vi "MarkedRobot.vi"(9 "id":u32, 10 "IA State Input":T2={"our_robots"=[], "enemy_robots"=[], "balls"=[], "geometry"={"line_width"=0, "field_length"=0, "field_width"=0, "boundary_width"=0, "referee_width"=0, "goal_width"=0, "goal_depth"=0, "goal_wall_width"=0, "center_circle_radius"=0, "defense_radius"=0, "defense_stretch"=0, "free_kick_from_defense_dist"=0, "penalty_spot_from_field_line_dist"=0, "penalty_line_from_spot_dist"=0}, "IA Judge"={"stage"="", "command"="", "our_goalie_id"=0.0, "enemy_goalie_id"=0.0, "command enum"=enum."Halt", "Time"=enum."Azul"}, "Received Timestamp"=timestamp(0 s since 1904-01-01), "Events"={"Touch"=FALSE, "Ball out"=FALSE, "id touch"=0.0, "Ball out of \nVision"=FALSE, "Ball inside \nGoalie area"=FALSE, "Robot not responding"=FALSE, "Robots responding status"=[1.0, 1.0, 1.0, 1.0, 1.0, 1.0], "Enemy Ball \nPossession"=FALSE, "Pass State"=FALSE, "id end of pass"=0.0, "Kick"=FALSE, "Id ini Possession"=0.0, "Ball Possesion"=FALSE, "Id Possesion"=0.0, "Direct Kick"=FALSE, "2nd Strk Ativo"=FALSE}}, 11 "AI Parameters":T1={"GotoKick"={"Dist do cone a frente"=150.0, "attacker farback"=1500.0, "Perto"=300.0, "min dist to kick"=150.0, "kick eps"=0.0, "Time to transition"=0.05}, "Attacker"={"CC chute"=0.09, "CC passe"=0.045, "Kick Force"=100.0, "ball-robot Kick"=200.0, "ball-robot Pass"=0.3, "drible\nAttk"=FALSE}, "Defender"={"D max"=1700.0, "Vel p/ robô av"=1000.0, "Kick Force"=100.0, "D atk-def"=0.0, "D farback"=0.0, "drible\ndef"=FALSE, "drible\ngoalie"=FALSE}, "Timeout"={"Field/v in x"=6.0, "Dist Robots"=300, "Dist up in y"=300}, "Pose Striker"={"dist"=200.0, "Numeric"=-4.0, "dist 2"=200.0, "drible\nstriker"=FALSE}, "Dist Stop"=300.0, "D ball out"=200, "D central gap "=150.0, "T pass"=0.0, "Force ++"=0.0, "range kick"=0.0, "Chute alto"=TRUE, "Marcador novo"=TRUE, "drible"=FALSE, "D drible"=300.0, "Versão Striker"=enum."3", "Defesa"=enum."ManMark", "Marcador"=enum."Marcar Segndo mais perigoso", "Receptor passe"=enum."2nd Striker", "Área"=enum."Quadrada"} {"D drible" format="%#_13g"; "D central gap" format="%#_13g"; "Dist Stop" format="%#_13g"; "Pose Striker"."Numeric" format="%#_13g"; "Defender"."Kick Force" format="%#_13g"; "Defender"."Vel p/ robô av" format="%#_13g"; "Attacker"."ball-robot Kick" format="%#_13g"; "Attacker"."Kick Force" format="%#_13g"; "Attacker"."CC passe" format="%#_13g"; "Attacker"."CC chute" format="%#_13g"; "GotoKick"."kick eps" format="%#_13g"; "GotoKick"."min dist to kick" format="%#_13g"; "GotoKick"."Perto" format="%#_13g"; "GotoKick"."attacker farback" format="%#_13g"; "GotoKick"."Dist do cone a frente" format="%#_13g"}) -> ()   [LabVIEW 2017]
uses:
  Core/AI Input.ctl
  Core/AI Robot.ctl
  Functions Enum.ctl
  AttackerStates.ctl
  Path Planning/RRT/PathDests.ctl
  Path Planning/RRT/PathDest.ctl
  Core/AI Ball.ctl
  Core/Field Size.ctl
  Core/AI Judge.ctl
  Command Enum.ctl
  Util/Events/Events.ctl
  AI Parameters.ctl
  d3ae8bea-2540-4cab-b848-3da8b8f91e54.vi
  <vilib>/Array/Sort 2D Array - Pop Stack.vi
  <vilib>/Array/Sort 2D Array - Push Stack.vi
panel:
  out "tempo para inimigo mais \npróximo da reta chegar a ela":dbl
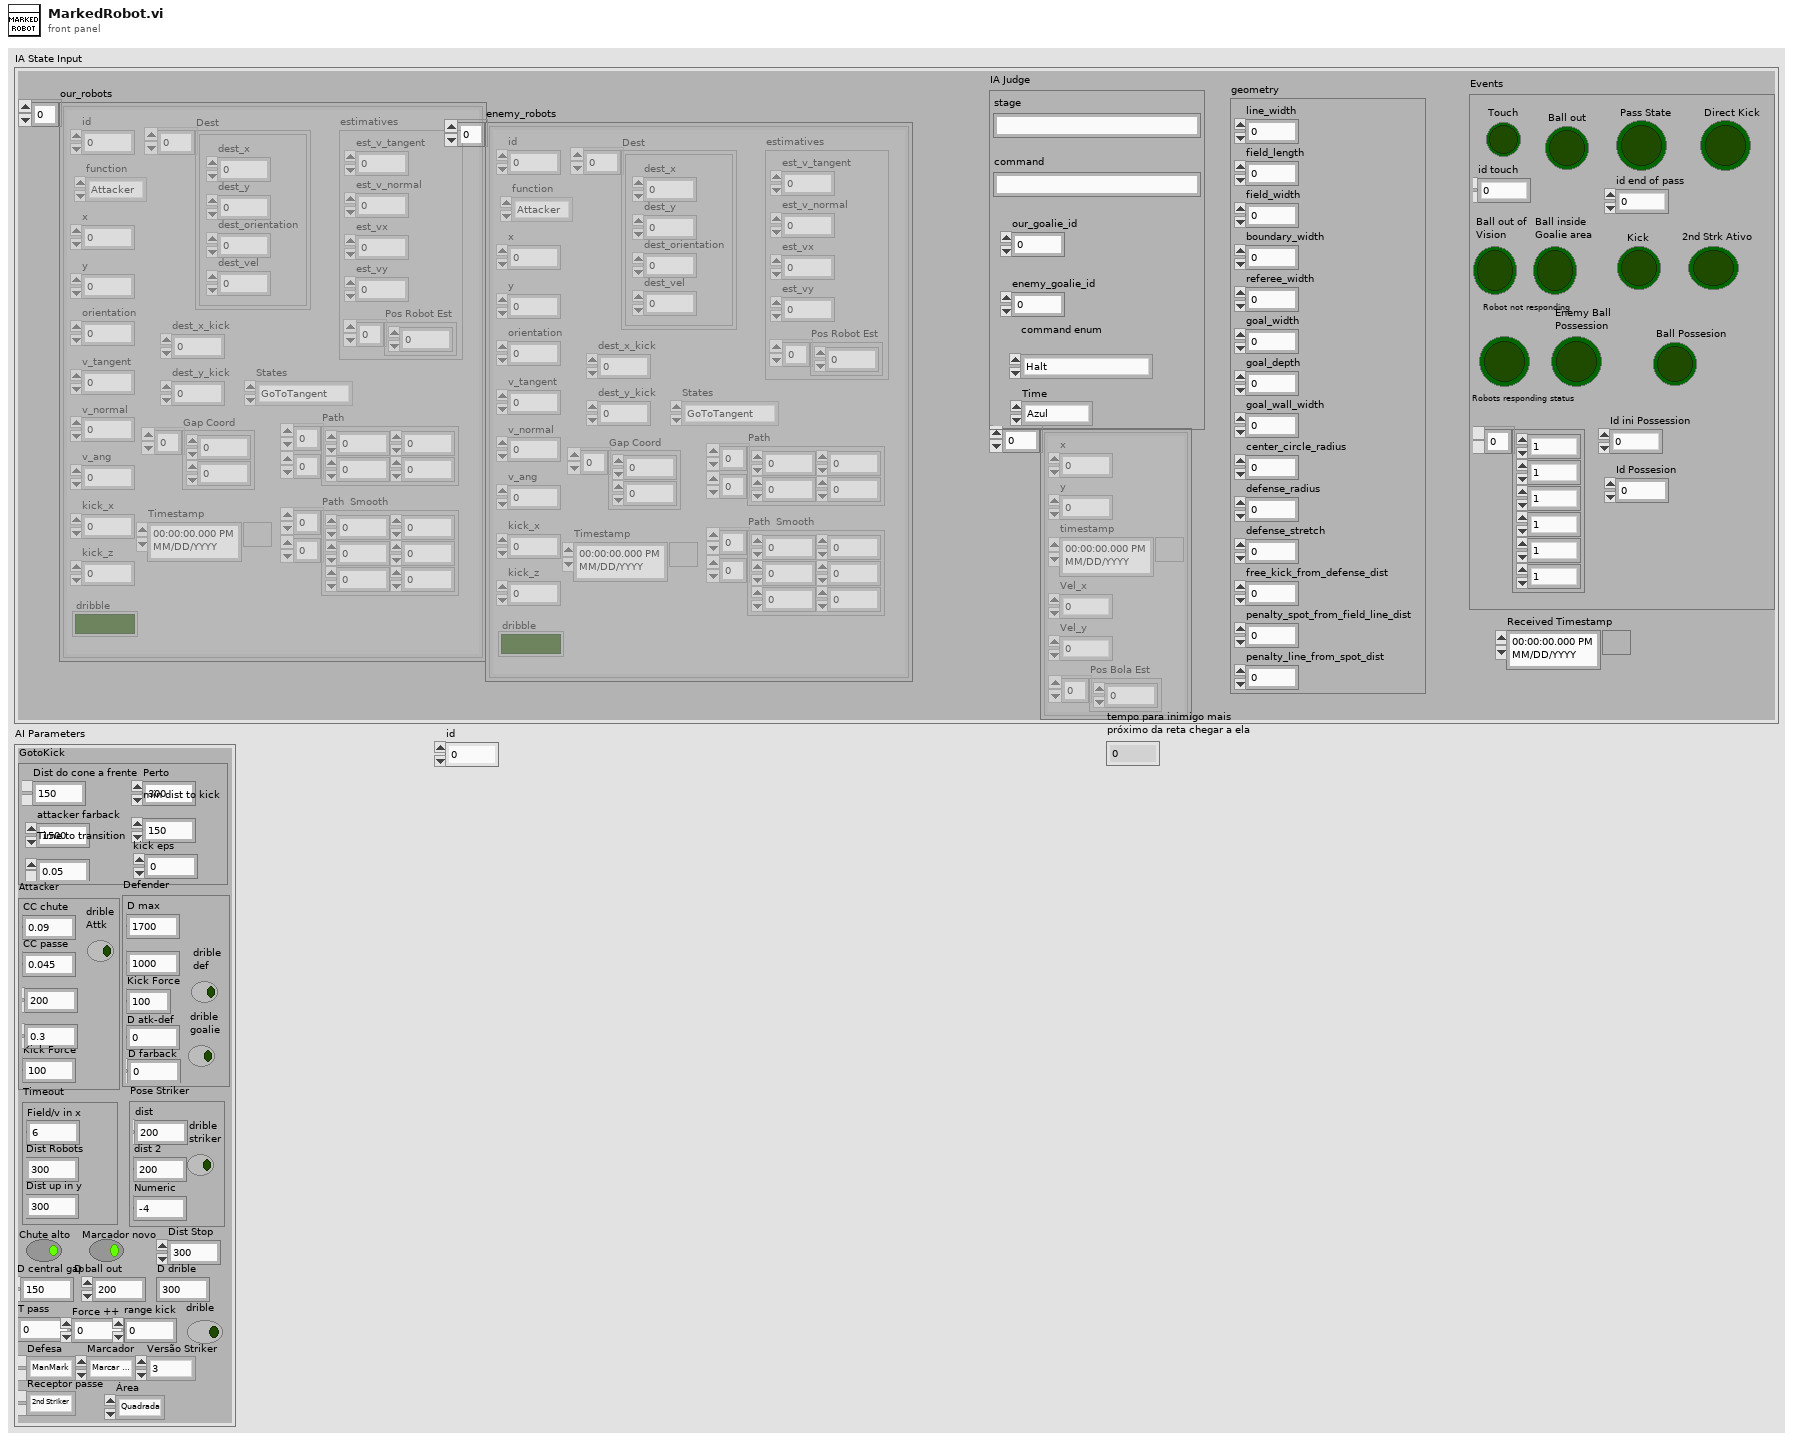
[diagram p1: front panel]
types:
  T1 = typedef "AI Parameters.ctl" = cluster{"GotoKick":cluster{"Dist do cone a frente":dbl, "attacker farback":dbl, "Perto":dbl, "min dist to kick":dbl, "kick eps":dbl, "Time to transition":dbl}, "Attacker":cluster{"CC chute":dbl, "CC passe":dbl, "Kick Force":dbl, "ball-robot Kick":dbl, "ball-robot Pass":dbl, "drible\nAttk":bool}, "Defender":cluster{"D max":dbl, "Vel p/ robô av":dbl, "Kick Force":dbl, "D atk-def":dbl, "D farback":dbl, "drible\ndef":bool, "drible\ngoalie":bool}, "Timeout":cluster{"Field/v in x":dbl, "Dist Robots":u32, "Dist up in y":u32}, "Pose Striker":cluster{"dist":dbl, "Numeric":dbl, "dist 2":dbl, "drible\nstriker":bool}, "Dist Stop":dbl, "D ball out":i32, "D central gap ":dbl, "T pass":dbl, "Force ++":dbl, "range kick":dbl, "Chute alto":bool, "Marcador novo":bool, "drible":bool, "D drible":dbl, "Versão Striker":enum16{"Auto", "3", "2", "1"}, "Defesa":enum16{"ManMark", "Barreira"}, "Marcador":enum16{"Marcar Segndo mais perigoso", "Marcar o mais perigoso"}, "Receptor passe":enum16{"Auto", "2nd Striker", "Striker"}, "Área":enum16{"Quadrada", "Circular"}}
  T2 = typedef "AI Input.ctl" = cluster{"our_robots":T3[], "enemy_robots":T3[], "balls":T8[], "geometry":T9, "IA Judge":T10, "Received Timestamp":timestamp, "Events":T12}
  T3 = typedef "AI Robot.ctl" = cluster{"id":u32, "function":T4, "x":dbl, "y":dbl, "orientation":dbl, "v_tangent":dbl, "v_normal":dbl, "v_ang":dbl, "kick_x":dbl, "kick_z":dbl, "dribble":bool, "Timestamp":timestamp, "estimatives":cluster{"est_v_tangent":dbl, "est_v_normal":dbl, "est_vx":dbl, "est_vy":dbl, "Pos Robot Est":dbl[]}, "dest_x_kick":dbl, "dest_y_kick":dbl, "Gap Coord":dbl[], "States":T5, "Path ":dbl[][], "Path  Smooth":dbl[][], "Dest":T6}
  T4 = typedef "Functions Enum.ctl" = enum16{"2nd Striker", "Attacker", "Goalie", "Defender", "Striker", "Goto 0", "Dummy", "Kicker", "ZigZag 0", "ZigZag 1", "ZigZag 2", "ZigZag 3", "ZigZag 4", "ZigZag 5", "ZigZag 6", "ZigZag 7", "ZigZag 8", ""}
  T5 = typedef "AttackerStates.ctl" = enum16{"Pass", "GoToTangent", "BallGetting", "GoToKick", ""}
  T6 = typedef "PathDests.ctl" = T7[]
  T7 = typedef "PathDest.ctl" = cluster{"dest_x":dbl, "dest_y":dbl, "dest_orientation":dbl, "dest_vel":dbl}
  T8 = typedef "AI Ball.ctl" = cluster{"x":dbl, "y":dbl, "timestamp":timestamp, "Vel_x":dbl, "Vel_y":dbl, "Pos Bola Est":dbl[]}
  T9 = typedef "Field Size.ctl" = cluster{"line_width":u32, "field_length":u32, "field_width":u32, "boundary_width":u32, "referee_width":u32, "goal_width":u32, "goal_depth":u32, "goal_wall_width":u32, "center_circle_radius":u32, "defense_radius":u32, "defense_stretch":u32, "free_kick_from_defense_dist":u32, "penalty_spot_from_field_line_dist":u32, "penalty_line_from_spot_dist":u32}
  T10 = typedef "AI Judge.ctl" = cluster{"stage":string, "command":string, "our_goalie_id":dbl, "enemy_goalie_id":dbl, "command enum":T11, "Time":enum16{"Azul", "Amarelo"}}
  T11 = typedef "Command Enum.ctl" = enum16{"Halt", "Stop", "Force Start", "PKA Normal Start", "Prepare Kickoff Ally", "PKE Normal Start", "Prepare Kickoff Enemy", "Prepare Penalty Ally", "PPA Normal Start", "Prepare Penalty Enemy", "PPE Normal Start", "Direct Free Enemy", "Direct Free Ally", "Indirect Free Enemy", "Indirect Free Ally", "Timeout Enemy", "Timeout Ally", "Goal Enemy", "Goal Ally", "Ball Placement Enemy", "Ball Placement Ally", "Normal Half Time", "Extra Time Break", "Extra Half Time", "None", "Post Game"}
  T12 = typedef "Events.ctl" = cluster{"Touch":bool, "Ball out":bool, "id touch":dbl, "Ball out of \nVision":bool, "Ball inside \nGoalie area":bool, "Robot not responding":bool, "Robots responding status":dbl[], "Enemy Ball \nPossession":bool, "Pass State":bool, "id end of pass":dbl, "Kick":bool, "Id ini Possession":dbl, "Ball Possesion":bool, "Id Possesion":dbl, "Direct Kick":bool, "2nd Strk Ativo":bool}
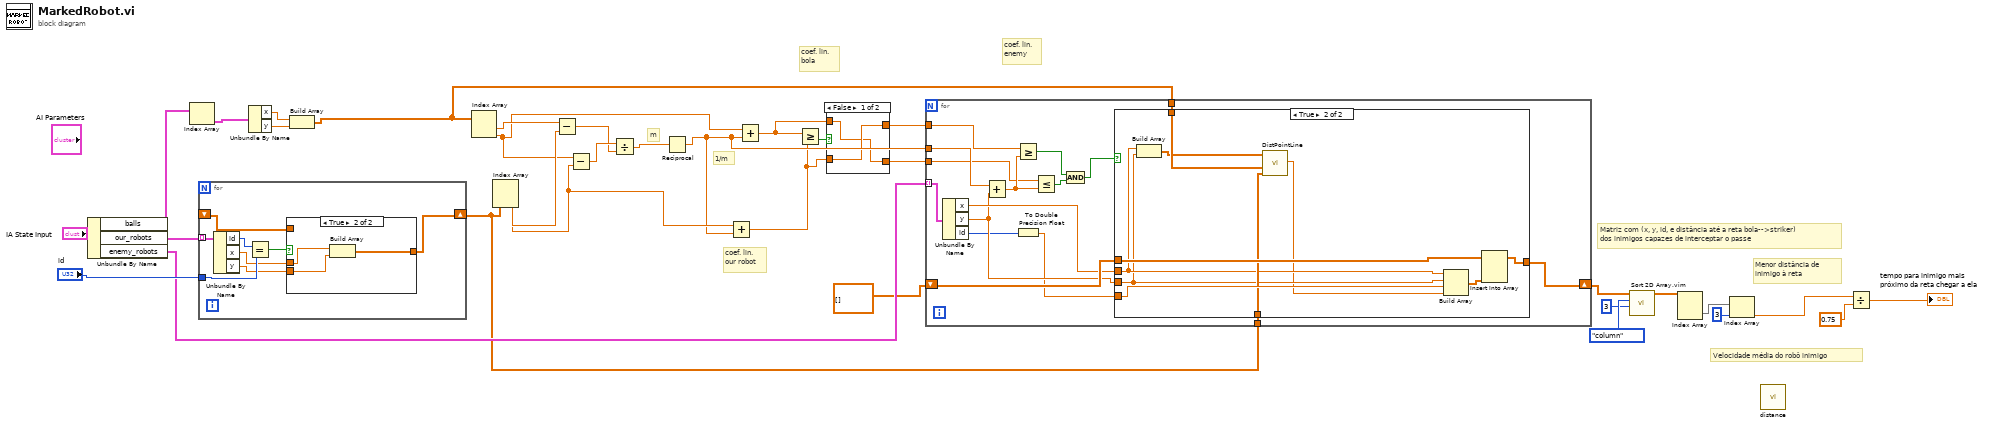
[diagram p0: block diagram]
diagram:
  # "Menor distância de \ninimigo à reta"
  # "Velocidade média do robô inimigo"
  # "Matriz com (x, y, id, e distância até a reta bola-->striker) \ndos inimigos capazes de interceptar o passe"
  # "coef. lin.\nbola"
  # "coef. lin.\nenemy"
  # "coef. lin.\nour robot"
  # "1/m"
  # "m"
  n1 = Unbundle By Name("IA State Input") -> ("balls"=w30:T8[], "our_robots"=w32:T3[], "enemy_robots"=w19:T3[])
  n2 = Index Array(array=w30) -> (element=w29:T8)  [unwired: 1 in]
  n3 = for {
    tunnel: w32 -> [w41] mode=indexing
    tunnel: "id" -> [w39]
    shift-right: [w35] -> w10
    shift-left: _ -> [w34]
    n4 = Unbundle By Name(w41) -> ("id"=w40:u32, "x"=w37:dbl, "y"=w36:dbl)
    n5 = Equal?(x=w40, y=w39) -> (x = y?=w38:bool)
    n6 = case shown="True" w38 {
      tunnel: w37 -> [_ w45]
      tunnel: w36 -> [_ w44]
      tunnel: [w42 w43] -> w35
      tunnel: w34 -> [w42 _]
      frame False {
      }
      frame True {
        n7 = Build Array(w45, w44) -> (w43:dbl[])
      }
    }
  }
  n8 = Unbundle By Name(w29) -> ("x"=w28:dbl, "y"=w27:dbl)
  n9 = Build Array(w28, w27) -> (w11:dbl[])
  n10 = Index Array(array=w11) -> (element #1=w26:dbl, element #2=w23:dbl)  [unwired: 2 in]
  n11 = Index Array(array=w10) -> (element #1=w25:dbl, element #2=w22:dbl)  [unwired: 2 in]
  n12 = Subtract(x=w26, y=w25) -> (x-y=w20:dbl)
  n13 = Subtract(x=w23, y=w22) -> (x-y=w21:dbl)
  n14 = Divide(x=w21, y=w20) -> (x/y=w24:dbl)
  n15 = Reciprocal(x=w24) -> (1/x=w18:dbl)
  n16 = Add(x=w22, y=w18) -> (x+y=w15:dbl)
  n17 = Add(x=w23, y=w18) -> (x+y=w16:dbl)
  n18 = Greater Or Equal?(x=w16, y=w15) -> (x >= y?=w17:bool)
  n19 = case shown="False" w17 {
    tunnel: [w47 w49] -> w14
    tunnel: w16 -> [w46 w49]
    tunnel: [w46 w48] -> w13
    tunnel: w15 -> [w47 w48]
    frame False {
    }
    frame True {
    }
  }
  n20 = for {
    tunnel: w19 -> [w65] mode=indexing
    tunnel: w18 -> [w64]
    shift-right: [w62] -> w6
    shift-left: dbl[][] [] -> [w63]
    tunnel: w14 -> [w57]
    tunnel: w13 -> [w56]
    tunnel: w11 -> [w51]
    tunnel: w10 -> [w50]
    n21 = Unbundle By Name(w65) -> ("x"=w55:dbl, "y"=w54:dbl, "id"=w53:u32)
    n22 = Add(x=w64, y=w54) -> (x+y=w61:dbl)
    n23 = Greater Or Equal?(x=w57, y=w61) -> (x >= y?=w59:bool)
    n24 = To Double Precision Float(number=w53) -> (double precision float=w52:dbl)
    n25 = Less Or Equal?(x=w56, y=w61) -> (x <= y?=w60:bool)
    n26 = And(x=w59, y=w60) -> (x .and. y?=w58:bool)
    n27 = case shown="True" w58 {
      tunnel: w63 -> [w66 w76]
      tunnel: [w66 w75] -> w62
      tunnel: w55 -> [_ w70]
      tunnel: w54 -> [_ w69]
      tunnel: w52 -> [_ w74]
      tunnel: w51 -> [_ w72]
      tunnel: w50 -> [_ w71]
      frame False {
      }
      frame True {
        n28 = Build Array(w70, w69) -> (w68:dbl[])
        n29 = call "DistPointLine.vi"("P2"=w71, "P1"=w72, "Q"=w68) -> ("distance"=w67:dbl)  [unwired: 8 in]
        n30 = Build Array(w70, w69, w74, w67) -> (w73:dbl[])
        n31 = Insert Into Array(array=w76, new element=w73) -> (w75:dbl[][])  [unwired: 2 in]
      }
    }
  }
  n32 = call "Sort 2D Array.vim"("index"=3, "dimension to index (column)"=enum16{"column", "row"}."column", "2D array"=w6) -> ("sorted 2D array"=w5:dbl[][])  [unwired: 7 in, 1 out]
  n33 = Index Array(array=w5) -> (element=w4:dbl[])  [unwired: 2 in]
  n34 = Index Array(array=w4, index=3) -> (element=w2:dbl)
  n35 = call "distance.vi"() -> ()  [unwired: 11 in, 1 out]
  n36 = Divide(x=w2, y=0.75) -> (x/y=→"tempo para inimigo mais \npróximo da reta chegar a ela":dbl)
